vi "EX_CP2112_GetDeviceMap.vi"() -> ()   [LabVIEW 2014]
uses:
  LV-CP2112_2014/LVProject/private/CP2112_QueueStatus.ctl
  LV-CP2112_2014/LVProject/private/CP2112_device.ctl
  LV-CP2112_2014/LVProject/private/CP2112_SMBUS_S0.ctl
panel:
  in  "btn_Quit":bool
  in  "scanRange(7bit)":cluster{"startRegistor":u8, "endRegistor":u8}={"startRegistor"=1, "endRegistor"=127} {"endRegistor" format="%.0x"; "startRegistor" format="%02x"}
  out "scanRange(8bit)":cluster{"startRegistor":u8, "endRegistor":u8}={"startRegistor"=0, "endRegistor"=255} {"endRegistor" format="%.0x"; "startRegistor" format="%02x"}
  out "RegistorMap":string[][](array[string])
  out "LaspedTime":u32
  in  "btn_Reset":bool
  in  "btn_Connect":bool
  in  "Connection":u16(ring) items=["ABC"]
  # "0     　1     　2     　3     　4    　 5      6     　7     　8     　 9    　 A     　B      C     　D     　E    　F"
  # "00\n10\n20\n30\n40\n50\n60\n70"
  # "[msec]"
  # "I2Cの接続状況をスキャンしてマップ表示します。\nラズベリーパイ等で、OS側ツール機能として提供されているものを\nCP2112で実現してみました。"
  # "I2Cのスレーブアドレスは7bitです。しかし、LSBにR/Wbitを加えて8bitで扱います。\nCP2112は8bitでスレーブアドレスを扱いますのでR/Wbit分のシフトをしています。"
  # "【使い方】\n①アプリケーションを起動します。\n②PCに接続されているCP2112を選択します。(Connectionリストから選択)\n③接続(Connect)します。スレーブアドレスをスキャンして反応があったアドレスを\n　表示します。()内のHex文字列がCP2112で使用するスレーブアドレスです。"
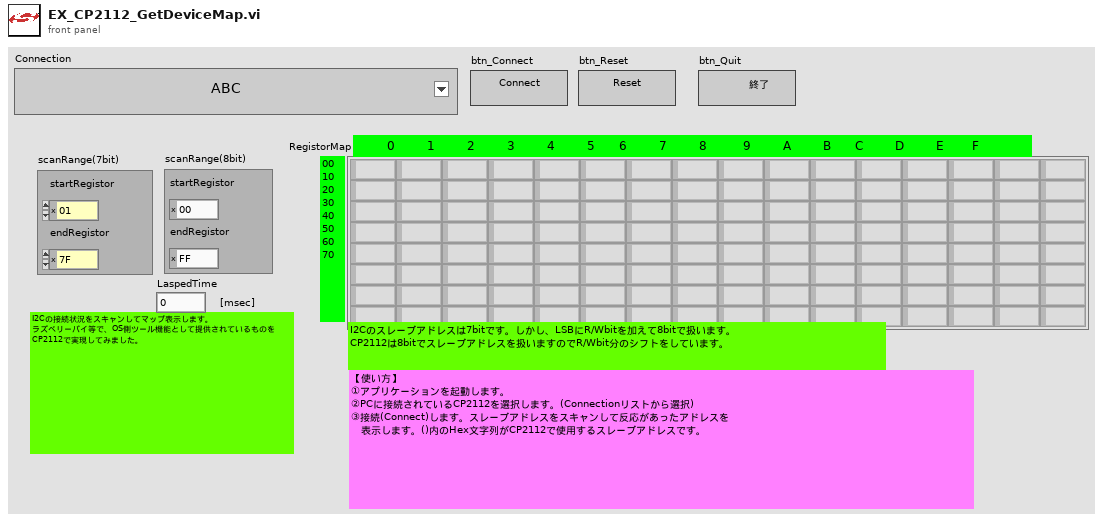
[diagram p1: front panel]
types:
  T1 = typedef "CP2112_device.ctl" = i32
  T2 = typedef "CP2112_QueueStatus.ctl" = enum16{"idle", "quit", "open", "close", "makeList", "reset", "getGPIO", "setGPIO", "readGPIO", "writeGPIO"}
  T3 = typedef "CP2112_SMBUS_S0.ctl" = enum8{"HID_SMBUS_S0_IDLE", "HID_SMBUS_S0_BUSY", "HID_SMBUS_S0_COMPLETE", "HID_SMBUS_S0_ERROR"}
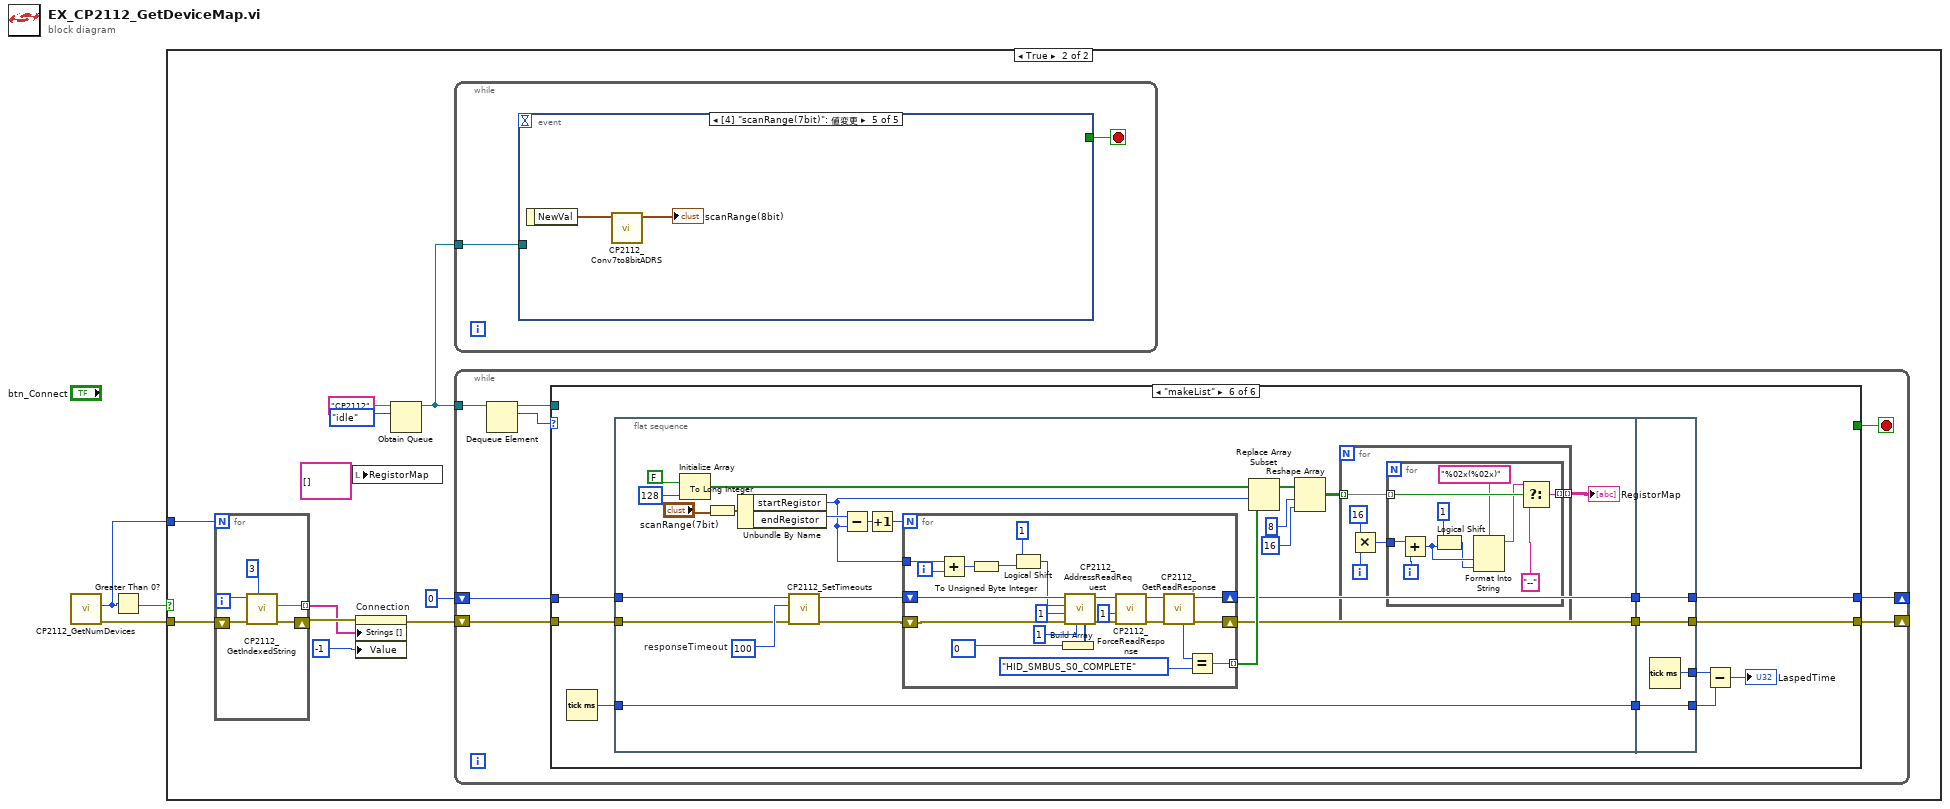
[diagram p0: block diagram]
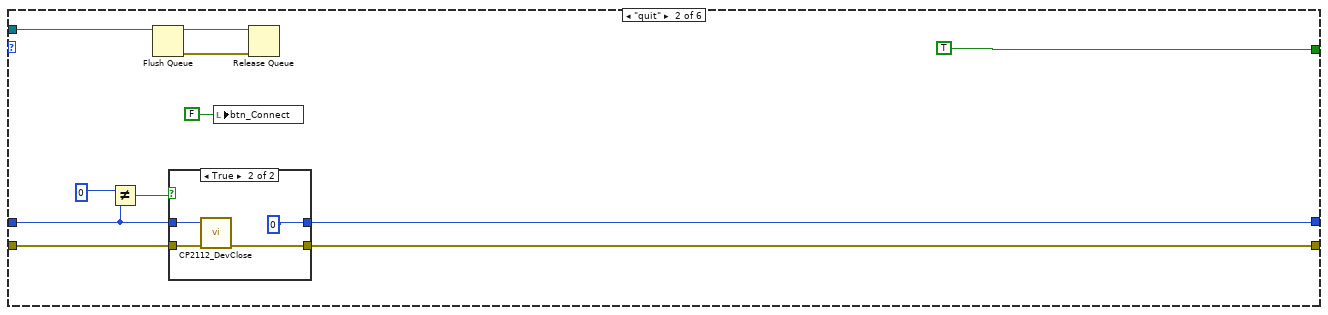
[diagram p4: hidden frame]
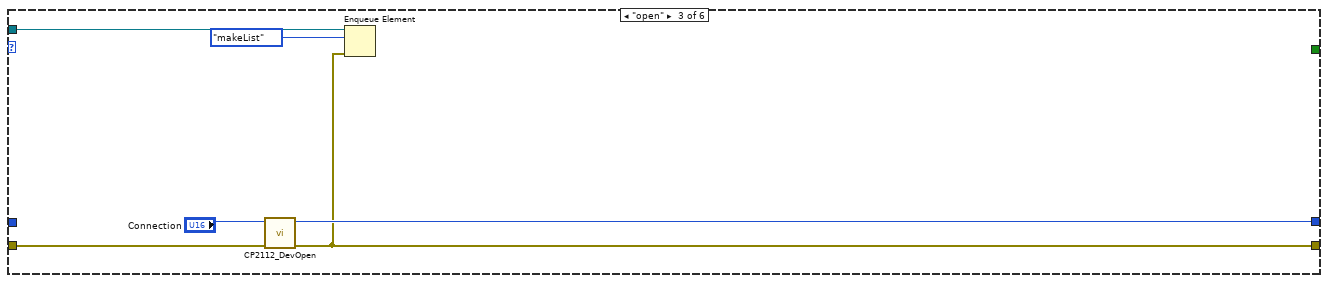
[diagram p6: hidden frame]
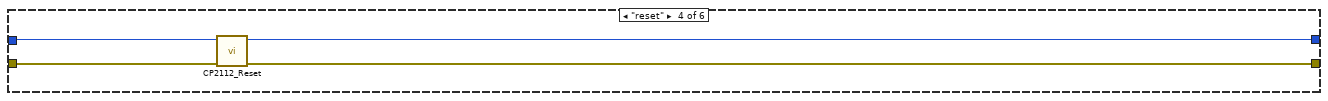
[diagram p7: hidden frame]
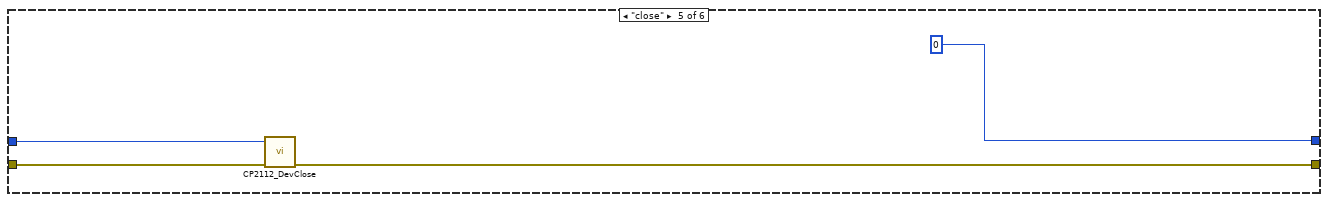
[diagram p8: hidden frame]
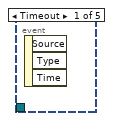
[diagram p9: hidden frame]
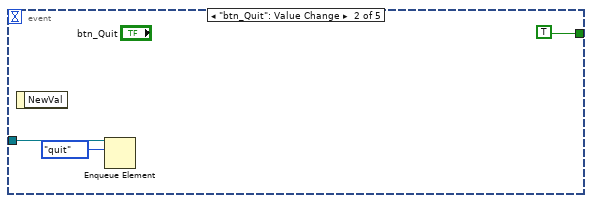
[diagram p10: hidden frame]
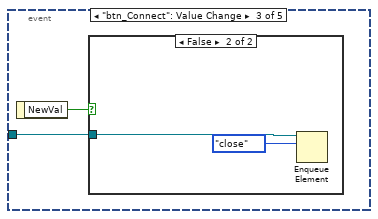
[diagram p11: hidden frame]
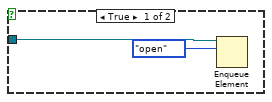
[diagram p12: hidden frame]
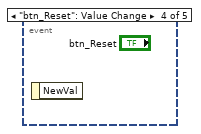
[diagram p13: hidden frame]
diagram:
  n1 = call "CP2112_GetNumDevices.vi"() -> ("error out"=w3:errorcluster, "numDevices"=w1:i32)  [unwired: 9 in, 1 out]
  n2 = Greater Than 0?(x=w1) -> (x > 0?=w2:bool)
  n3 = case shown="TRUE" w2 {
    tunnel: w3 -> [_ w9]
    tunnel: w1 -> [_ w8]
    frame False {
    }
    frame True {
      n4 = for {
        N: w8 -> [_]
        shift-right: [w16] -> w6
        shift-left: w9 -> [w19]
        tunnel: [w15] -> w5 mode=indexing
        i -> [w18]
        n5 = call "CP2112_GetIndexedString.vi"("options"=3, "error in (no error)"=w19, "DevicesNum"=w18) -> ("error out"=w16:errorcluster, "deviceString"=w15:string)  [unwired: 6 in, 1 out]
      }
      n6 = local write "RegistorMap"(string[][] [] ("RegistorMap")) -> ()
      n7 = property on="Connection" class="Ring （指定）"(error in=w6, "Strings []"=w5, "Value"=-1) -> (error out=w7:errorcluster)  [unwired: 1 in, 1 out]
      n8 = Obtain Queue(name (unnamed)="CP2112" ("名前（名前なし）"), element data type=CP2112_QueueStatus."idle") -> (queue out=w12:refnum<queue>)  [unwired: 3 in, 2 out]
      n9 = while {
        tunnel: w12 -> [w136]
        stop <- w137 stop-if-true
        n10 = event shown="[4] \"scanRange(7bit)\": 値変更" {
          selector: _ -> [_ _ _ _ _]
          dyn-events: _ -> [_ _ _ _ _]
          timeout: _ -> [_ _ _ _ _]
          tunnel: [_ TRUE _ _ _] -> w137
          tunnel: w136 -> [_ w139 w141 _ _]
          event Timeout {
            n11 = event-data() -> ()  [unwired: 1 in, 3 out]
          }
          event "btn_Quit": Value Change {
            n12 = event-data() -> ()  [unwired: 1 in, 1 out]
            n13 = Enqueue Element(queue=w139, element=CP2112_QueueStatus."quit" ("要素")) -> ()  [unwired: 2 in, 3 out]
          }
          event "btn_Connect": Value Change {
            n14 = event-data() -> ("NewVal"=w142:bool)  [unwired: 1 in]
            n15 = case shown="FALSE" w142 {
              tunnel: w141 -> [w144 w146]
              frame True {
                n16 = Enqueue Element(queue=w144, element=CP2112_QueueStatus."open" ("要素")) -> ()  [unwired: 2 in, 3 out]
              }
              frame False {
                n17 = Enqueue Element(queue=w146, element=CP2112_QueueStatus."close" ("要素")) -> ()  [unwired: 2 in, 3 out]
              }
            }
          }
          event "btn_Reset": Value Change {
            n18 = event-data() -> ()  [unwired: 1 in, 1 out]
          }
          event "scanRange(7bit)": Value Change {
            n19 = event-data() -> ("NewVal"=w147:cluster{"startRegistor":u8, "endRegistor":u8})  [unwired: 1 in]
            n20 = call "CP2112_Conv7to8bitADRS.vi"("7bitAdress"=w147) -> ("8bitAddressOut"=→"scanRange(8bit)":cluster{"startRegistor":u8, "endRegistor":u8})  [unwired: 10 in]
          }
        }
      }
      n21 = while {
        tunnel: w12 -> [w27]
        shift-right: [w22] -> _
        shift-left: w7 -> [w23]
        shift-right: [w21] -> _
        shift-left: T1 0 ("device") -> [w20]
        stop <- w24 stop-if-true
        n22 = Dequeue Element(queue=w27) -> (queue out=w26:refnum<queue>, element=w25:T2)  [unwired: 2 in, 2 out]
        n23 = case shown="\"makeList\"" w25 {
          tunnel: w26 -> [_ w39 w50 _ _ _]
          tunnel: [_ TRUE _ _ _ _] -> w24
          tunnel: w23 -> [w28 w33 w52 w55 w59 w71]
          tunnel: [w29 w31 w51 w53 T1 0 ("device") w69] -> w21
          tunnel: [w28 w32 w48 w54 w58 w68] -> w22
          tunnel: w20 -> [w29 w35 _ w56 w60 w70]
          frame "idle", Default {
          }
          frame "quit" {
            n24 = Not Equal?(x=T1 0 ("device"), y=w35) -> (x != y?=w34:bool)
            n25 = Flush Queue(queue=w39) -> (queue out=w38:refnum<queue>, error out=w37:errorcluster)  [unwired: 1 in, 1 out]
            n26 = case shown="TRUE" w34 {
              tunnel: w35 -> [w42 w46]
              tunnel: w33 -> [w41 w45]
              tunnel: [w41 w44] -> w32
              tunnel: [w42 T1 0 ("device")] -> w31
              frame False {
              }
              frame True {
                n27 = call "CP2112_DevClose.vi"("error in (no error)"=w45, "device"=w46) -> ("error out"=w44:errorcluster)  [unwired: 9 in]
              }
            }
            n28 = local write "btn_Connect"(FALSE ("btn_Connect")) -> ()
            n29 = Release Queue(queue=w38, error in (no error)=w37) -> ()  [unwired: 1 in, 3 out]
          }
          frame "open" {
            n30 = call "CP2112_DevOpen.vi"("error in (no error)"=w52, "deviceNum"="Connection") -> ("error out"=w48:errorcluster, "device"=w51:T1)  [unwired: 7 in, 1 out]
            n31 = Enqueue Element(queue=w50, element=CP2112_QueueStatus."makeList" ("要素"), error in (no error)=w48) -> ()  [unwired: 1 in, 3 out]
          }
          frame "reset" {
            n32 = call "CP2112_Reset.vi"("error in (no error)"=w55, "device"=w56) -> ("error out"=w54:errorcluster, "deviceOut"=w53:T1)  [unwired: 7 in, 1 out]
          }
          frame "close" {
            n33 = call "CP2112_DevClose.vi"("error in (no error)"=w59, "device"=w60) -> ("error out"=w58:errorcluster)  [unwired: 9 in]
          }
          frame "makeList" {
            n34 = Tick Count (ms)() -> (millisecond timer value=w67:u32)
            n35 = flat-sequence {
              tunnel: w71 -> [w77]
              tunnel: w70 -> [w76]
              tunnel: w67 -> [w72]
              tunnel: [w75] -> w66
              tunnel: [w73] -> w65
              tunnel: [w72] -> w64
              tunnel: [w133] -> w63
              tunnel: [w134] -> w68
              tunnel: [w135] -> w69
              tunnel: w66 -> [w135]
              tunnel: w65 -> [w134]
              tunnel: w64 -> [w133]
              tunnel: [w132] -> w62
              frame #0 {
                w94 = u32 100  # responseTimeout
                n36 = Initialize Array(FALSE, 128 ("次元サイズ")) -> (w81:bool[])
                n37 = To Long Integer(number="scanRange(7bit)") -> (32bit integer=w88:cluster{"startRegistor":i32, "endRegistor":i32})
                n38 = Unbundle By Name(w88) -> ("startRegistor"=w78:i32, "endRegistor"=w91:i32)
                n39 = call "CP2112_SetTimeouts.vi"("error in (no error)"=w77, "responseTimeout"=w94, "device"=w76) -> ("error out"=w74:errorcluster, "deviceOut"=w93:T1)  [unwired: 6 in, 1 out]
                n40 = Subtract(x=w91, y=w78) -> (x-y=w90:i32)
                n41 = Increment(x=w90) -> (x+1=w89:i32)
                n42 = for {
                  N: w89 -> [_]
                  shift-right: [w126] -> w75
                  shift-left: w93 -> [w127]
                  tunnel: w78 -> [w124]
                  tunnel: [w112] -> w80 mode=indexing
                  shift-right: [w110] -> w73
                  shift-left: w74 -> [w111]
                  i -> [w125]
                  n43 = Add(x=w124, y=w125) -> (x+y=w123:i32)
                  n44 = To Unsigned Byte Integer(number=w123) -> (unsigned 8bit integer=w116:u8)
                  n45 = Logical Shift(y=1, x=w116) -> (x << y=w115:u8)
                  n46 = Build Array(u8 0 ("targetAddressSize")) -> (w120:u8[])
                  n47 = call "CP2112_AddressReadRequest.vi"("targetAddress[]"=w120, "targetAddressSize"=u8 1, "error in (no error)"=w111, "numByteToRead"=i16 1, "slaveAddress"=w115, "device"=w127) -> ("error out"=w130:errorcluster, "deviceOut"=w131:T1)  [unwired: 3 in, 1 out]
                  n48 = call "CP2112_ForceReadResponse.vi"("error in (no error)"=w130, "numByteToRead"=i16 1, "device"=w131) -> ("error out"=w129:errorcluster, "deviceOut"=w128:T1)  [unwired: 6 in, 1 out]
                  n49 = call "CP2112_GetReadResponse.vi"("error in (no error)"=w129, "device"=w128) -> ("error out"=w110:errorcluster, "deviceOut"=w126:T1, "HID_SMBUS_S0"=w113:T3)  [unwired: 4 in, 3 out]
                  n50 = Equal?(x=w113, y=CP2112_SMBUS_S0."HID_SMBUS_S0_COMPLETE" ("HID_SMBUS_S0")) -> (x = y?=w112:bool)
                }
                n51 = Replace Array Subset(array=w81, new element=w80, index=w78) -> (w79:bool[])
                n52 = Reshape Array(w79, 8 ("次元サイズ"), 16 ("次元サイズ")) -> (w85:bool[][])
                n53 = for {
                  tunnel: w85 -> [w99] mode=indexing
                  tunnel: [w98] -> w84 mode=indexing
                  i -> [w97]
                  n54 = Multiply(x=16, y=w97) -> (x*y=w95:i32)
                  n55 = for {
                    tunnel: w99 -> [w109] mode=indexing
                    tunnel: [w107] -> w98 mode=indexing
                    tunnel: w95 -> [w105]
                    i -> [w106]
                    n56 = Add(x=w105, y=w106) -> (x+y=w101:i32)
                    n57 = Logical Shift(y=1, x=w101) -> (x << y=w100:i32)
                    n58 = Format Into String(format string="%02x(%02x)" ("形式文字列"), w101, w100) -> (resulting string=w104:string)  [unwired: 2 in, 1 out]
                    n59 = Select(t=w104, s=w109, f="--") -> (s? t:f=w107:string)
                  }
                }
                "RegistorMap" <- w84
              }
              frame #1 {
                n60 = Tick Count (ms)() -> (millisecond timer value=w132:u32)
              }
            }
            n61 = Subtract(x=w62, y=w63) -> (x-y=→"LaspedTime":u32)
          }
        }
      }
    }
  }
